vi "Read Projects.vi"(8 "error in (no error)":errorcluster, 11 "Projects in":refnum<class "Projects.lvclass">) -> (0 "error out":errorcluster, 2 "Projects":map{string, T1}(c390), 3 "Projects out":refnum<class "Projects.lvclass">)   [LabVIEW 2020, in "Projects.lvclass"]
uses:
  Projects.lvclass
  Projects.lvclass/Projects.ctl
  Controls/Project Info.ctl
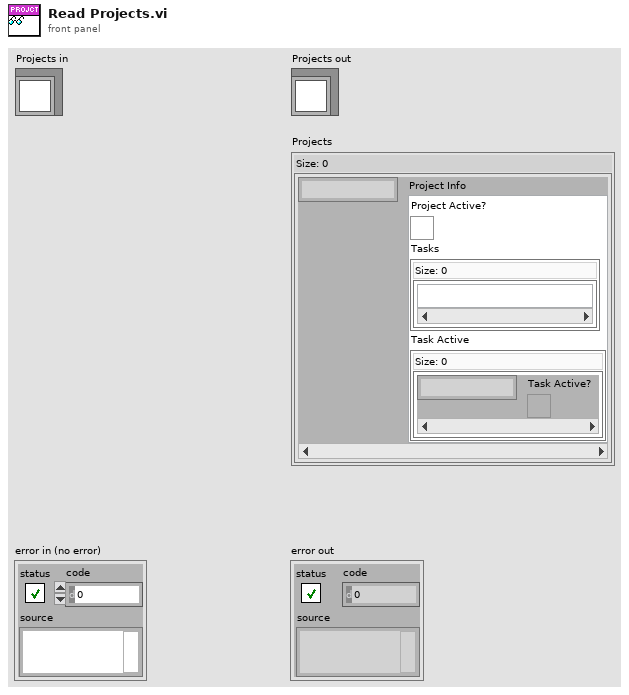
[diagram p1: front panel]
types:
  T1 = typedef "Project Info.ctl" = cluster{"Project Active?":bool, "Tasks":set{string}, "Task Active":map{string, bool}}
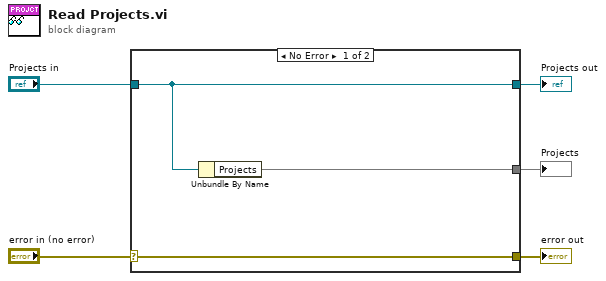
[diagram p0: block diagram]
diagram:
  n1 = case shown="No Error" "error in (no error)" {
    selector: "error in (no error)" -> [w8 w9]
    tunnel: [w8 w9] -> w4
    tunnel: [w7 w10] -> w2
    tunnel: "Projects in" -> [w7 w10]
    tunnel: [w6 _] -> w1
    frame No Error {
      n2 = Unbundle By Name(w7) -> ("Projects"=w6:map{string, T1})
    }
    frame Error {
    }
  }
  "error out" <- w4
  "Projects out" <- w2
  "Projects" <- w1
